vi "PXI Global Data Notifier.vi"(11 "error in (no error)":errorcluster) -> (6 "AI Waveforms":dbl[][](array[numeric]), 10 "Waveform Graph":dbl[][](graph), 15 "error out":errorcluster)   [LabVIEW 2015]
uses:
  DAQ Engine VIs/PXI Globals.vi
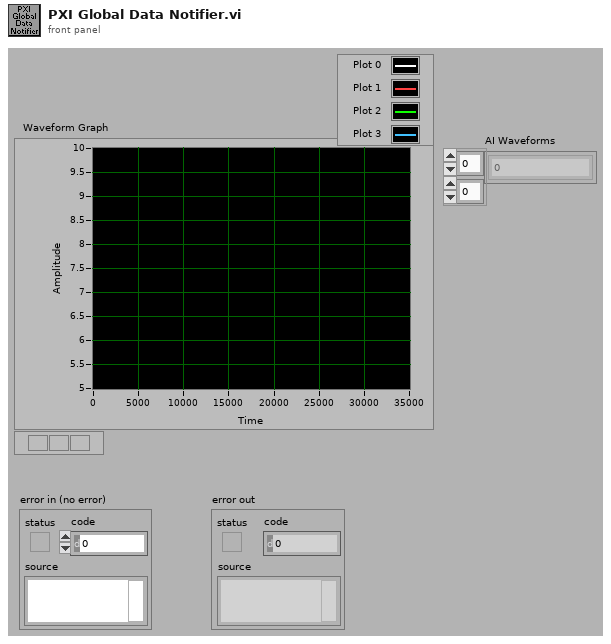
[diagram p1: front panel]
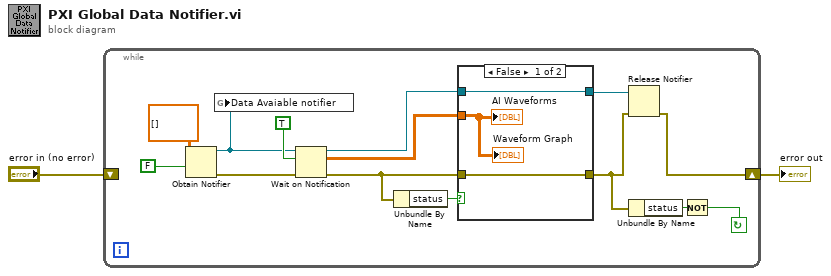
[diagram p0: block diagram]
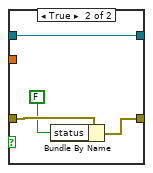
[diagram p2: hidden frame]
diagram:
  n1 = while {
    shift-right: [w3] -> w1
    shift-left: "error in (no error)" -> [_]
    stop <- w11 continue-if-true
    n2 = Obtain Notifier(notification data type=dbl[][] [] ("AI Waveforms 2"), create if not found? (T)=FALSE) -> (notifier out=w7:refnum<notifier>, error out=w8:errorcluster)  [unwired: 2 in, 1 out]
    n3 = global write "PXI Globals.vi" "Data Avaiable notifier"(w7) -> ()
    n4 = Wait on Notification(notifier=w7, ignore previous (F)=TRUE, error in (no error)=w8) -> (notifier out=w6:refnum<notifier>, notification=w12:dbl[][], error out=w16:errorcluster)  [unwired: 1 in, 1 out]
    n5 = Unbundle By Name(w16) -> ("status"=w15:bool)
    n6 = case shown="False" w15 {
      tunnel: [w19 w22] -> w4
      tunnel: w16 -> [w19 w23]
      tunnel: w12 -> [w18 _]
      tunnel: [w17 w20] -> w5
      tunnel: w6 -> [w17 w20]
      frame False {
        "AI Waveforms" <- w18
        "Waveform Graph" <- w18
      }
      frame True {
        n7 = Bundle By Name(cluster=w23, "status"=FALSE) -> (w22:errorcluster)
      }
    }
    n8 = Release Notifier(notifier=w5, error in (no error)=w4) -> (error out=w3:errorcluster)  [unwired: 1 in, 2 out]
    n9 = Unbundle By Name(w4) -> ("status"=w14:bool)
    n10 = Not(x=w14) -> (.not. x?=w11:bool)
  }
  "error out" <- w1
